vi "SPITest.vi"() -> ()   [LabVIEW 2013]
uses:
  <vilib>/Rock Robotics/SystemInterfaces/DIO/FPGA_DIOChannel.ctl
  <vilib>/Rock Robotics/WPI/SPI/WPI_SPIBits Per Word.ctl
  <vilib>/Rock Robotics/SystemInterfaces/DIO/FPGA_DIOPWMChannel.ctl
panel:
  out "error out 9":errorcluster
  out "error out 8":errorcluster
  in  "Value 2":u8
  out "error out 7":errorcluster
  in  "Value":bool
  out "error out 6":errorcluster
  out "error out 5":errorcluster
  out "error out 4":errorcluster
  out "error out 3":errorcluster
  out "error out 2":errorcluster
  out "Received Data":u32
  out "error out":errorcluster
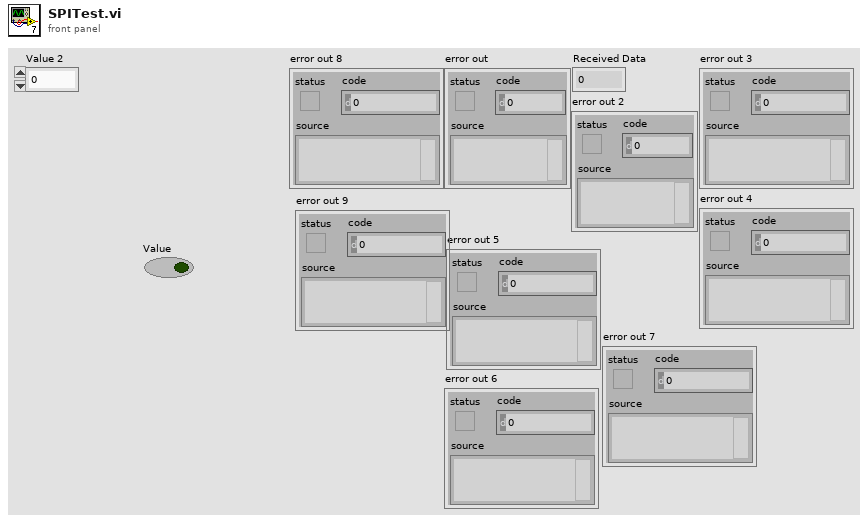
[diagram p1: front panel]
types:
  T1 = typedef "FPGA_DIOChannel.ctl" = enum8{"DIO 1", "DIO 2", "DIO 3", "DIO 4", "DIO 5", "DIO 6", "DIO 7", "DIO 8", "DIO 9", "DIO 10", "DIO 11", "DIO 12", "DIO 13", "DIO 14", "Invalid"}
  T2 = typedef "WPI_SPIBits Per Word.ctl" = u8
  T3 = typedef "WPI_DigitalOutputDevRef.ctl" = cluster{"Digital Module":T4, "DIO Channel":T1, "DevStatus":errorcluster}
  T4 = typedef "FPGA_TypedefDigitalModule.ctl" = enum16{"Digital Module 1", "Digital Module 2"}
  T5 = typedef "WPI_DigitalInputDevRef.ctl" = cluster{"DevStatus":errorcluster, "DIO Channel":T1, "Digital Module":T4}
  T6 = typedef "WPI_SPIDevRef.ctl" = cluster{"DevStatus":errorcluster}
  T7 = typedef "FPGA_DIOPWMChannel.ctl" = enum8{"PWM 1", "PWM 2", "PWM 3", "PWM 4", "PWM 5", "PWM 6", "PWM 7", "PWM 8", "PWM 9", "PWM 10", "Invalid"}
  T8 = typedef "WPI_PWMDeviceRef.ctl" = cluster{"DeviceStatus":errorcluster, "Digital Module":T4, "PWM Channel":T7}
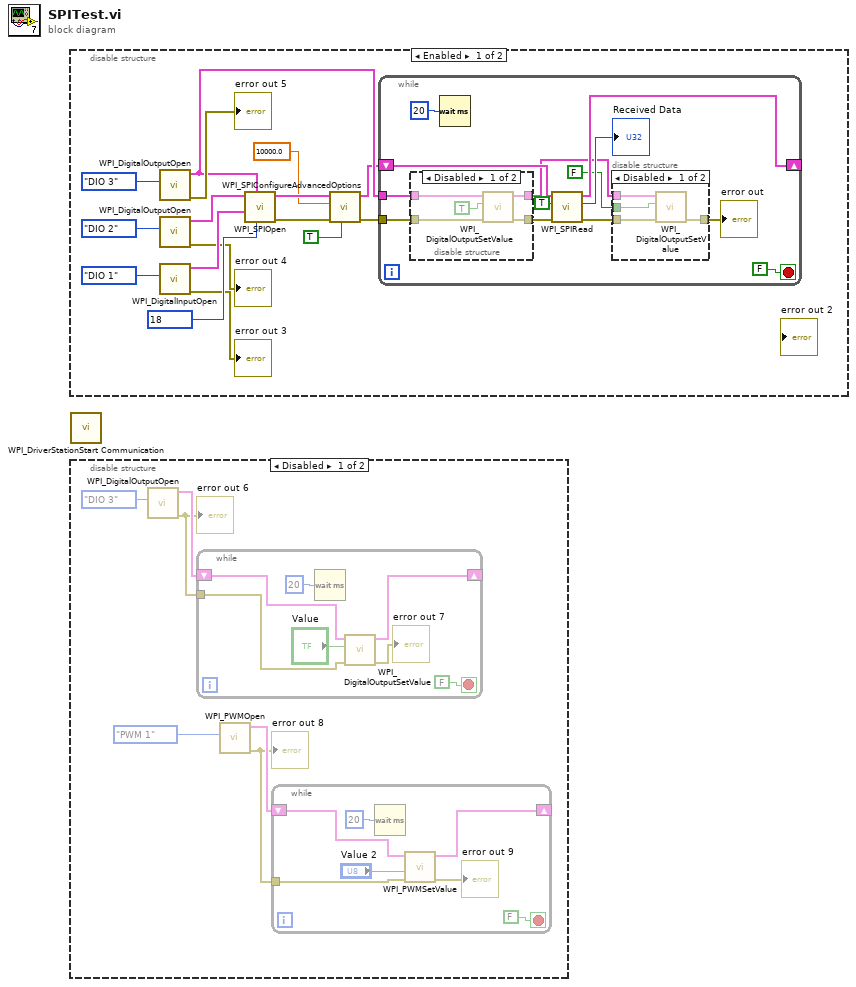
[diagram p0: block diagram]
diagram:
  n1 = disable-structure shown="Enabled" {
    frame Enabled {
      w11 = T2 18 items=["8-Bit"=8, "16-Bit"=16, "32-Bit"=32] ("Bits Per Word")
      n2 = call <vilib>:"WPI_DigitalOutputOpen.vi"("DIO Channel"=FPGA_DIOChannel."DIO 3") -> ("error out"=→"error out 5":errorcluster, "DigitalOutputDevRef"=w7:T3)  [unwired: 9 in]
      n3 = call <vilib>:"WPI_DigitalOutputOpen.vi"("DIO Channel"=FPGA_DIOChannel."DIO 2") -> ("error out"=→"error out 4":errorcluster, "DigitalOutputDevRef"=w14:T3)  [unwired: 9 in]
      n4 = call <vilib>:"WPI_DigitalInputOpen.vi"("DIO Channel"=FPGA_DIOChannel."DIO 1") -> ("error out"=→"error out 3":errorcluster, "DigitalInputDevRef"=w12:T5)  [unwired: 9 in]
      n5 = call <vilib>:"WPI_SPIOpen.vi"("Bits Per Word"=w11, "Chip Select"=w7, "Master-In Slave-Out"=w12, "Clock"=w14) -> ("error out"=w3:errorcluster, "SPIDevRef"=w6:T6)  [unwired: 6 in]
      n6 = call <vilib>:"WPI_SPIConfigureAdvancedOptions.vi"("Clock Phase (Data On Falling) (F)"=TRUE, "error in (no error)"=w3, "Clock Rate (Hz)"=10000.0, "SPIDevRef"=w6) -> ("error out"=w5:errorcluster, "SPIDevRef"=w4:T6)  [unwired: 6 in]
      n7 = while {
        shift-right: [w25] -> _
        shift-left: w4 -> [w27]
        tunnel: w7 -> [w24]
        tunnel: w5 -> [w23]
        stop <- FALSE stop-if-true
        n8 = disable-structure shown="Disabled" {
          disable-tunnel: w24 -> [w38 _]
          disable-tunnel: w23 -> [w37 _]
          disable-tunnel: [w36 _] -> w22
          disable-tunnel: [w35 _] -> w19
          frame Disabled {
            n9 = call <vilib>:"WPI_DigitalOutputSetValue.vi"("error in (no error)"=w37, "Value"=TRUE, "DigitalOutputDevRef"=w38) -> ("error out"=w36:errorcluster, "DigitalOutputDevRef"=w35:T3)  [unwired: 7 in]
          }
          frame Enabled {
          }
        }
        n10 = Wait (ms)(milliseconds to wait=u32 20) -> ()  [unwired: 1 out]
        n11 = call <vilib>:"WPI_SPIRead.vi"("error in (no error)"=w22, "Initiate Transfer (F)"=TRUE, "SPIDevRef"=w27) -> ("error out"=w21:errorcluster, "Received Data"=→"Received Data":u32, "SPIDevRef"=w25:T6)  [unwired: 6 in]
        n12 = disable-structure shown="Disabled" {
          disable-tunnel: w21 -> [w33 _]
          disable-tunnel: [w32 _] -> w20
          disable-tunnel: w19 -> [w31 _]
          disable-tunnel: FALSE ("Value") -> [w30 _]
          frame Disabled {
            n13 = call <vilib>:"WPI_DigitalOutputSetValue.vi"("error in (no error)"=w33, "Value"=w30, "DigitalOutputDevRef"=w31) -> ("error out"=w32:errorcluster)  [unwired: 7 in, 1 out]
          }
          frame Enabled {
          }
        }
        "error out" <- w20
      }
    }
    frame Disabled {
    }
  }
  n14 = call <vilib>:"WPI_DriverStationStart Communication.vi"() -> ()  [unwired: 12 in]
  n15 = disable-structure shown="Disabled" {
    frame Disabled {
      n16 = call <vilib>:"WPI_DigitalOutputOpen.vi"("DIO Channel"=FPGA_DIOChannel."DIO 3") -> ("error out"=w42:errorcluster, "DigitalOutputDevRef"=w43:T3)  [unwired: 9 in]
      "error out 6" <- w42
      n17 = while {
        tunnel: w42 -> [w57]
        shift-right: [w52] -> _
        shift-left: w43 -> [w58]
        stop <- FALSE stop-if-true
        n18 = Wait (ms)(milliseconds to wait=u32 20) -> ()  [unwired: 1 out]
        n19 = call <vilib>:"WPI_DigitalOutputSetValue.vi"("error in (no error)"=w57, "Value"="Value", "DigitalOutputDevRef"=w58) -> ("error out"=→"error out 7":errorcluster, "DigitalOutputDevRef"=w52:T3)  [unwired: 7 in]
      }
      n20 = call <vilib>:"WPI_PWMOpen.vi"("PWM Channel"=FPGA_DIOPWMChannel."PWM 1") -> ("error out"=w39:errorcluster, "PWMDeviceRef"=w40:T8)  [unwired: 9 in]
      "error out 8" <- w39
      n21 = while {
        shift-right: [w48] -> _
        shift-left: w40 -> [w49]
        tunnel: w39 -> [w46]
        stop <- FALSE stop-if-true
        n22 = Wait (ms)(milliseconds to wait=u32 20) -> ()  [unwired: 1 out]
        n23 = call <vilib>:"WPI_PWMSetValue.vi"("error in (no error)"=w46, "Value"="Value 2", "PWMDeviceRef"=w49) -> ("error out"=→"error out 9":errorcluster, "PWMDeviceRef"=w48:T8)  [unwired: 7 in]
      }
    }
    frame Enabled {
    }
  }
